vi "B12dll.vi"(8 "error in (no error)":errorcluster, 10 "z":dbl[](array[numeric]), 11 "t":dbl) -> (0 "error out":errorcluster, 3 "b out":dbl)   [LabVIEW 2016]
doc: "subroutine B12 (t,z,b)\n\ncompute b12 as a function of temperature and composition.\n\nINPUTS:\n t--temperature [K]\n z--composition [array of mol frac]\nOUTPUTS:\n b--b12 [(L/mol)^2]"
uses:
  REFPROP.DLL
panel:
  # "REFPROP-B12dll.vi"
  # "void  B12dll(double *t, double *z, double *b);"
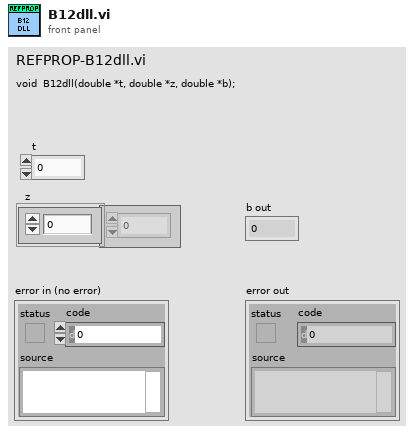
[diagram p1: front panel]
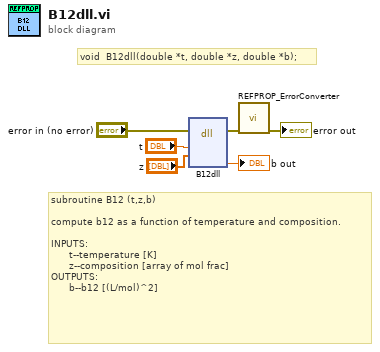
[diagram p0: block diagram]
diagram:
  # "void  B12dll(double *t, double *z, double *b);"
  # "subroutine B12 (t,z,b)\n\ncompute b12 as a function of temperature and composition.\n\nINPUTS:\n      t--temperature [K]\n      z--composition [array of mol frac]\nOUTPUTS:\n      b--b12 [(L/mol)^2]"
  n1 = dll-call lib="S:/009 - Testing/02 - Performance Testing/REFPROP/REFPROP.*" fn="B12dll"(error in="error in (no error)", "t"="t", "z"="z") -> (error out=w3:errorcluster, "b"=→"b out":dbl)  [unwired: 6 in, 1 out]
  n2 = call "REFPROP_ErrorConverter.vi"("error in (no error)"=w3) -> ("error out"=→"error out":errorcluster)  [unwired: 10 in]
